vi "SelectColor.vi"(2 "CMF":dbl[][](array[numeric]), 3 "Illuminant":cluster{"String":string, "Array":dbl[]}, 4 "Selected RGB":string(combo)) -> (0 "Reflectance":dbl[](array[numeric]), 1 "Color,XYZ,RGB,Lab":T1)   [LabVIEW 2013]
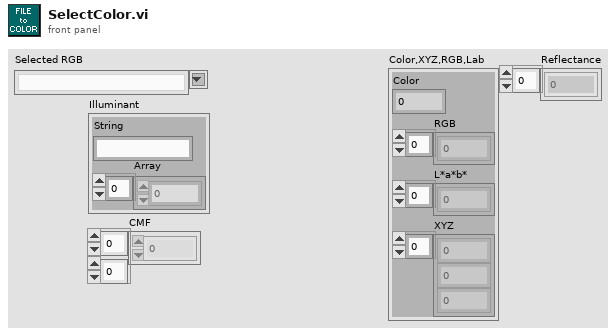
[diagram p1: front panel]
types:
  T1 = cluster{"Color":u32, "RGB":dbl[], "L*a*b*":dbl[], "XYZ":dbl[]}
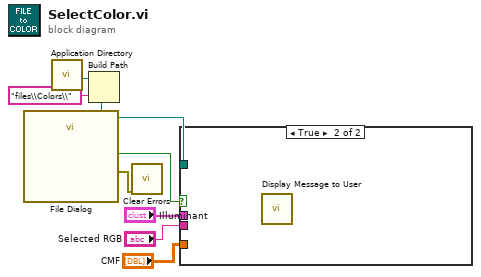
[diagram p0: block diagram]
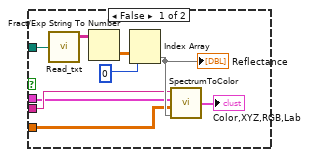
[diagram p2: hidden frame]
diagram:
  n1 = call <vilib>:"Application Directory.vi"() -> ("Application Directory"=w8:path)
  n2 = Build Path(base path=w8, name or relative path="files\\Colors\\") -> (appended path=w7:path)
  n3 = call "File Dialog"("start path"=w7) -> ("selected path"=w5:path, "cancelled"=w6:bool, "error out"=w4:errorcluster)  [unwired: 11 in, 1 out]
  n4 = call <vilib>:"Clear Errors.vi"("error in (no error)"=w4) -> ()  [unwired: 6 in, 1 out]
  n5 = case shown="True" w6 {
    tunnel: w5 -> [w15 _]
    tunnel: "CMF" -> [w13 _]
    tunnel: "Selected RGB" -> [w12 _]
    tunnel: "Illuminant" -> [w11 _]
    frame False {
      n6 = call "Read_txt.vi"("file path (dialog if empty)"=w15) -> ("Elements"=w18:string[][])  [unwired: 2 out]
      n7 = Fract/Exp String To Number(string=w18) -> (number=w17:dbl[][])  [unwired: 3 in, 1 out]
      n8 = Index Array(array=w17, index (col)=0 ("index (row)")) -> (element=w14:dbl[])  [unwired: 1 in]
      "Reflectance" <- w14
      n9 = call "SpectrumToColor.vi"("Reflectance"=w14, "CMF"=w13, "Illuminant"=w11, "Selected RGB"=w12) -> ("Color,XYZ,RGB,Lab"=→"Color,XYZ,RGB,Lab":T1)
    }
    frame True {
      n10 = call "Display Message to User"() -> ()  [unwired: 10 in, 2 out]
    }
  }
